vi "Read FunctionReturn.vi"(8 "error in (no error)":errorcluster, 11 "MatlabExperiment in":refnum<class "MatlabExperiment.lvclass">) -> (0 "error out":errorcluster, 2 "FunctionReturn":cluster{"Name":string, "Data":variant}[](array[cluster]), 3 "MatlabExperiment out":refnum<class "MatlabExperiment.lvclass">)   [LabVIEW 2014, in "AcquisitionCoreObjects.lvlib" / "MatlabExperiment.lvclass"]
uses:
  MatlabExperiment.lvclass
  MatlabExperiment.lvclass/MatlabExperiment.ctl
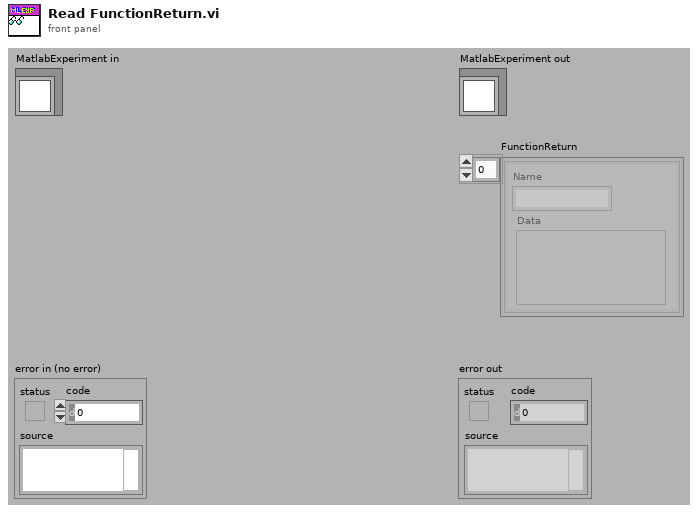
[diagram p1: front panel]
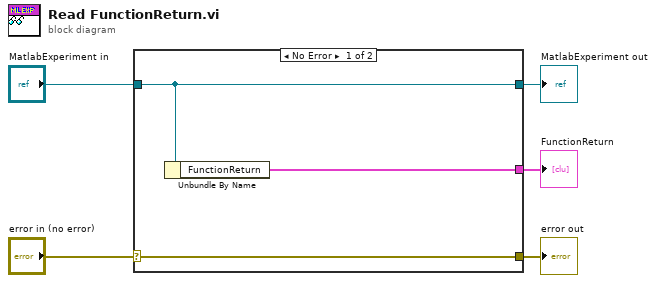
[diagram p0: block diagram]
diagram:
  n1 = case shown="No Error" "error in (no error)" {
    selector: "error in (no error)" -> [w8 w9]
    tunnel: [w8 w9] -> w4
    tunnel: [w7 w10] -> w2
    tunnel: "MatlabExperiment in" -> [w7 w10]
    tunnel: [w6 _] -> w1
    frame No Error {
      n2 = Unbundle By Name(w7) -> ("FunctionReturn"=w6:cluster{"Name":string, "Data":variant}[])
    }
    frame Error {
    }
  }
  "error out" <- w4
  "MatlabExperiment out" <- w2
  "FunctionReturn" <- w1
